vi "Get_VI_printed_page_orientation.vi"(0 "reference in":refnum<vi>, 1 "error in (no error)":errorcluster) -> (2 "reference out":refnum<vi>, 3 "Orientaion":T1 items=["Unchanged", "portrait", "landscape"], 4 "error out":errorcluster)   [LabVIEW 2020, in "NI_ReportGenerationCore.lvlib"]
uses:
  <vilib>/Utility/NIReport.llb/NI_ReportGenerationCore.lvlib
  <vilib>/printing/EasyPrintingControls.llb/orientation.ctl
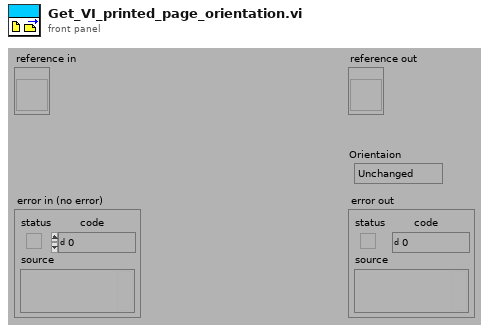
[diagram p1: front panel]
types:
  T1 = typedef "NI_ReportGenerationCore.lvlib/orientation.ctl" = u16
  T2 = enum32{"Portrait", "Landscape", "Rotated Portrait", "Rotated Landscape"}
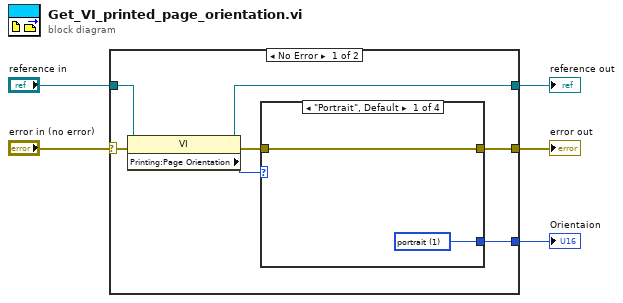
[diagram p0: block diagram]
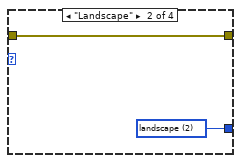
[diagram p2: hidden frame]
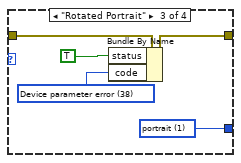
[diagram p3: hidden frame]
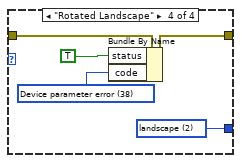
[diagram p4: hidden frame]
diagram:
  n1 = case shown="No Error" "error in (no error)" {
    selector: "error in (no error)" -> [w12 w28]
    tunnel: [w9 w28] -> w4
    tunnel: "reference in" -> [w8 w27]
    tunnel: [w7 w27] -> w2
    tunnel: [w6 _] -> w1
    frame No Error {
      n2 = property class="VI"(reference=w8, error in=w12) -> (reference out=w7:refnum<vi>, error out=w10:errorcluster, "Printing:Page Orientation"=w11:T2)
      n3 = case shown="\"Portrait\", Default" w11 {
        tunnel: [w14 w16 w21 w26] -> w6
        tunnel: w10 -> [w13 w15 w20 w23]
        tunnel: [w13 w15 w17 w22] -> w9
        frame "Portrait", Default {
          w14 = T1 1 items=["Unchanged", "portrait", "landscape"] ("orientation (unchanged)")
        }
        frame "Landscape" {
          w16 = T1 2 items=["Unchanged", "portrait", "landscape"] ("orientation (unchanged)")
        }
        frame "Rotated Portrait" {
          w18 = 38 items=["No error", "Argument error", "Memory is full", "Out of zone", "End of file", "File already open", "Generic file I/O error", "File not found", "File permission error", "Disk is full", "Duplicate path", "Too many files open", "System feature not enabled", "Resource file not found", "Cannot add resource", "Resource not found", "Image not found", "Image memory error", "Pen does not exist", "Config type invalid", "Config token not found", "Config parse error", "Config memory error", "Bad external code format", "Bad external code offset", "External code not present", "Null window", "Destroy window error", "Null menu", "Print aborted", "Bad print record", "Print driver error", "Windows error during printing", "Memory error during printing", "Print dialog error", "Generic print error", "Invalid device refnum", "Device not found", "Device parameter error", "Device unit error", "Cannot open device", "Device call aborted", "Generic error", "Cancelled by user", "Object ID too low", "Object ID too high", "Object not in heap", "Unknown heap", "Unknown object (invalid DefProc)", "Unknown object (DefProc not in table)", "Message out of range", "Invalid (null) method", "Unknown message", "Manager call not supported", "Bad address", "Network operation in progress", "Network operation timed out", "Connection is busy", "Network attribute not supported", "Network error", "Address in use", "System out of memory", "Connection aborted", "Connection refused", "Not connected", "Already connected", "Connection closed", "Initialization error (interapplication manager)", "Bad occurrence", "Wait on unbound occurrence handler", "Occurrence queue overflow", "Datalog type conflict", "Unused", "Unrecognized type (interapplication manager)", "Memory corrupt", "Failed to make temporary DLL", "Old CIN version", "Drag socket not found", "Failed to load drop-object", "Failed to register OLE object", "Failed to release OLE object", "Format specifier type mismatch", "Unknown format specifier", "Too few format specifiers", "Too many format specifiers", "Scan failed", "Newer CIN version", "Error converting to variant", "Runtime menu error", "Password tampered", "Variant attribute not found", "Incompatible variant data type", "Event data is not available", "Event Store is not present", "Occurrence is not found", "Event Queue is not created", "Event info is not available", "Refnum passed is NULL", "Error retrieving Class GUID", "Error retrieving CoClass GUID", "Error retrieving TypeLib GUID.", "Bad built application magic bytes.", "Specific driver is different from the specific driver associated with the Logical Name.", "There is no session opened to the class driver.", "Max Error", "MAX - Error with config objects", "MAX - Error loading configuration", "MAX - Group not supported", "Singlecast connections can not send to multicast addresses.", "Multicast connections can not send to singlecast addresses.", "Specified IP address not in multicast address range.", "Attempt to write to read-only multicast connection.", "Attempt to read from write-only multicast connection."]
          w21 = T1 1 items=["Unchanged", "portrait", "landscape"] ("orientation (unchanged)")
          n4 = Bundle By Name(cluster=w20, "status"=TRUE, "code"=w18) -> (w17:errorcluster)
        }
        frame "Rotated Landscape" {
          w24 = 38 items=["No error", "Argument error", "Memory is full", "Out of zone", "End of file", "File already open", "Generic file I/O error", "File not found", "File permission error", "Disk is full", "Duplicate path", "Too many files open", "System feature not enabled", "Resource file not found", "Cannot add resource", "Resource not found", "Image not found", "Image memory error", "Pen does not exist", "Config type invalid", "Config token not found", "Config parse error", "Config memory error", "Bad external code format", "Bad external code offset", "External code not present", "Null window", "Destroy window error", "Null menu", "Print aborted", "Bad print record", "Print driver error", "Windows error during printing", "Memory error during printing", "Print dialog error", "Generic print error", "Invalid device refnum", "Device not found", "Device parameter error", "Device unit error", "Cannot open device", "Device call aborted", "Generic error", "Cancelled by user", "Object ID too low", "Object ID too high", "Object not in heap", "Unknown heap", "Unknown object (invalid DefProc)", "Unknown object (DefProc not in table)", "Message out of range", "Invalid (null) method", "Unknown message", "Manager call not supported", "Bad address", "Network operation in progress", "Network operation timed out", "Connection is busy", "Network attribute not supported", "Network error", "Address in use", "System out of memory", "Connection aborted", "Connection refused", "Not connected", "Already connected", "Connection closed", "Initialization error (interapplication manager)", "Bad occurrence", "Wait on unbound occurrence handler", "Occurrence queue overflow", "Datalog type conflict", "Unused", "Unrecognized type (interapplication manager)", "Memory corrupt", "Failed to make temporary DLL", "Old CIN version", "Drag socket not found", "Failed to load drop-object", "Failed to register OLE object", "Failed to release OLE object", "Format specifier type mismatch", "Unknown format specifier", "Too few format specifiers", "Too many format specifiers", "Scan failed", "Newer CIN version", "Error converting to variant", "Runtime menu error", "Password tampered", "Variant attribute not found", "Incompatible variant data type", "Event data is not available", "Event Store is not present", "Occurrence is not found", "Event Queue is not created", "Event info is not available", "Refnum passed is NULL", "Error retrieving Class GUID", "Error retrieving CoClass GUID", "Error retrieving TypeLib GUID.", "Bad built application magic bytes.", "Specific driver is different from the specific driver associated with the Logical Name.", "There is no session opened to the class driver.", "Max Error", "MAX - Error with config objects", "MAX - Error loading configuration", "MAX - Group not supported", "Singlecast connections can not send to multicast addresses.", "Multicast connections can not send to singlecast addresses.", "Specified IP address not in multicast address range.", "Attempt to write to read-only multicast connection.", "Attempt to read from write-only multicast connection."]
          w26 = T1 2 items=["Unchanged", "portrait", "landscape"] ("orientation (unchanged)")
          n5 = Bundle By Name(cluster=w23, "status"=TRUE, "code"=w24) -> (w22:errorcluster)
        }
      }
    }
    frame Error {
    }
  }
  "reference out" <- w2
  "error out" <- w4
  "Orientaion" <- w1
